vi "Initialize Com Port.vi"(8 "Error In":errorcluster, 11 "ECU COM Port":refnum<visa-resource-name>) -> (0 "Error Out":errorcluster, 3 "ECU COM Port Out":refnum<visa-resource-name>)   [LabVIEW 2017]
doc: "<b>Description</b>\nThis VI initializes the COM port.\n\n<b>Inputs</b>\nECU Com Port: The com port of the ECU.\n\n<b>Outputs</b>\nECU Com Port Out: The com port of the ECU."
uses:
  <vilib>/Instr/_visa.llb/VISA Configure Serial Port (Instr).vi
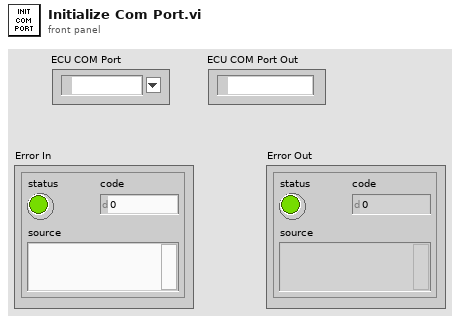
[diagram p1: front panel]
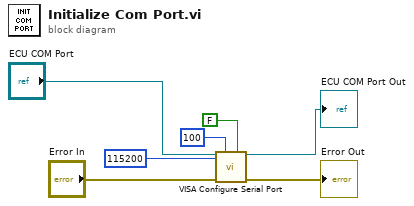
[diagram p0: block diagram]
diagram:
  n1 = call-poly "VISA Configure Serial Port"("VISA resource name"="ECU COM Port", "timeout (10sec)"=u32 100, "Enable Termination\nChar (T)"=FALSE ("Enable Termination\nChar (T)"), "baud rate (9600)"=u32 115200, "error in (no error)"="Error In") -> ("VISA resource name out"=→"ECU COM Port Out":refnum<visa-resource-name>, "error out"=→"Error Out":errorcluster)  [unwired: 9 in]
